vi "Constructor.vi"(8 "error in (no error)":errorcluster, 11 "Agilent 3458A in":refnum<class "Agilent 3458A.lvclass">) -> (0 "error out":errorcluster, 2 "Init":bool, 3 "Agilent 3458A out":refnum<class "Agilent 3458A.lvclass">)   [LabVIEW 2011, in "Agilent 3458A.lvclass"]
uses:
  Agilent 3458A.lvclass
  Agilent 3458A.lvclass/Agilent 3458A.ctl
  <instrlib>/Agilent 3458/Agilent 3458.lvlib
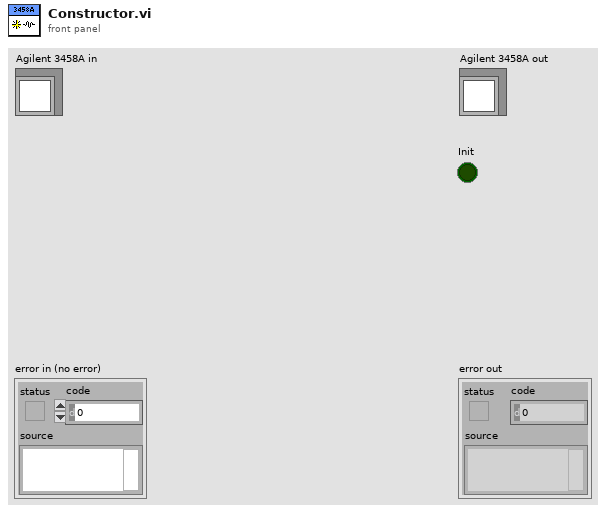
[diagram p1: front panel]
types:
  T1 = typedef "Agilent 3458A.lvclass/Measurement Configuration.ctl" = cluster{"Function":enum16{"DC Voltage", "AC Voltage", "AC + DC Voltage", "DC Current", "AC Current", "AC + DC Current", "2-Wire Resistance", "4-Wire Resistance", "Frequency", "Period", "Direct Sampling DC", "Direct Sampling AC", "Sub-Sampling DC", "Sub-Sampling AC"}, " Manual Resolution":enum16{"4.5", "5.5", "6.5", "7.5", "8.5"}, "Frequency Source":enum16{"AC + DC Current", "AC + DC Voltage", "AC Current", "AC Voltage"}, "Auto Range":enum16{"OFF", "ON", "ONCE"}}
  T2 = typedef "Agilent 3458A.lvclass/Measurement Integration.ctl" = cluster{"Power Line Cycles":dbl}
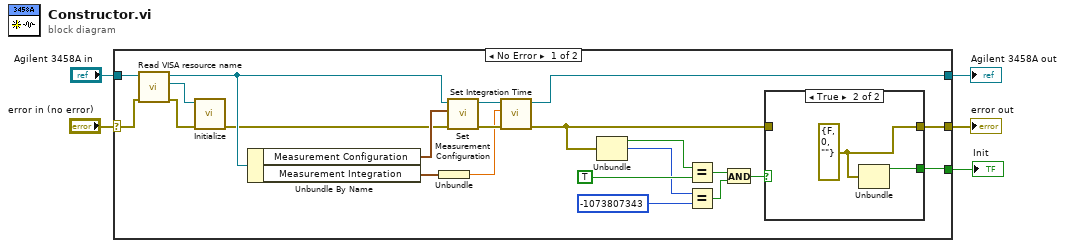
[diagram p0: block diagram]
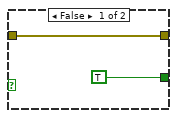
[diagram p2: hidden frame]
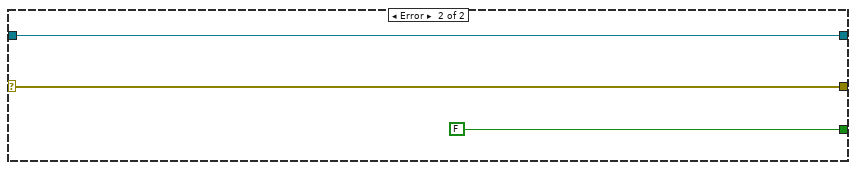
[diagram p3: hidden frame]
diagram:
  n1 = case shown="No Error" "error in (no error)" {
    selector: "error in (no error)" -> [w25 w34]
    tunnel: [w9 w34] -> w4
    tunnel: [w18 w33] -> w2
    tunnel: "Agilent 3458A in" -> [w27 w33]
    tunnel: [w6 FALSE] -> w1
    frame No Error {
      n2 = call-dynamic "Read VISA resource name.vi"("error in (no error)"=w25, "Multimeter in"=w27) -> ("error out"=w24:errorcluster, "VISA resource name"=w26:refnum<visa-resource-name>, "Multimeter out"=w22:refnum<class "Agilent 3458A.lvclass">)  [unwired: 7 in]
      n3 = call <instrlib>:"Initialize.vi"("error in (no error)"=w24, "VISA resource name"=w26) -> ("error out"=w21:errorcluster)  [unwired: 8 in, 1 out]
      n4 = Unbundle By Name(w22) -> ("Measurement Configuration"=w23:T1, "Measurement Integration"=w17:T2)
      n5 = Unbundle(w17) -> ("Power Line Cycles"=w16:dbl)
      n6 = call-dynamic "Set Measurement Configuration.vi"("error in (no error)"=w21, "Measurement Configuration"=w23, "Agilent 3458A in"=w22) -> ("error out"=w20:errorcluster, "Agilent 3458A out"=w19:refnum<class "Agilent 3458A.lvclass">)  [unwired: 7 in]
      n7 = call-dynamic "Set Integration Time.vi"("error in (no error)"=w20, "Integration Time"=w16, "Agilent 3458A in"=w19) -> ("error out"=w7:errorcluster, "Agilent 3458A out"=w18:refnum<class "Agilent 3458A.lvclass">)  [unwired: 7 in]
      n8 = Unbundle(w7) -> ("status"=w15:bool, "code"=w13:i32)  [unwired: 1 out]
      n9 = Equal?(x=w15, y=TRUE ("status")) -> (x = y?=w11:bool)
      n10 = Equal?(x=w13, y=-1073807343 ("code")) -> (x = y?=w10:bool)
      n11 = And(x=w11, y=w10) -> (x .and. y?=w8:bool)
      n12 = case shown="True" w8 {
        tunnel: [w29 w31] -> w9
        tunnel: w7 -> [w29 _]
        tunnel: [TRUE w30] -> w6
        frame False {
        }
        frame True {
          w31 = errorcluster {"status"=FALSE, "code"=0, "source"=""} ("error in (no error) 2")
          n13 = Unbundle(w31) -> ("status"=w30:bool)  [unwired: 2 out]
        }
      }
    }
    frame Error {
    }
  }
  "error out" <- w4
  "Agilent 3458A out" <- w2
  "Init" <- w1
